vi "Encode_Base64 (SubVI).vi"(8 "error in (no error)":errorcluster, 11 "File Path":path=path "C:/Users/Voodoo/Desktop/loc_eps_3dcartrot.gif") -> (0 "error out":errorcluster, 3 "Base 64":string)   [LabVIEW 2016]
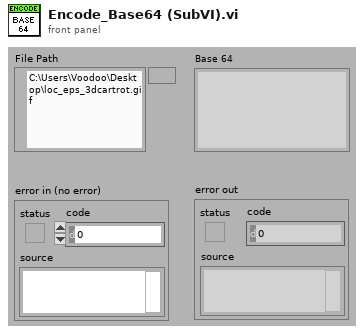
[diagram p1: front panel]
types:
  T1 = cluster{"unsigned byte array[0]":u8, "unsigned byte array[1]":u8, "unsigned byte array[2]":u8}
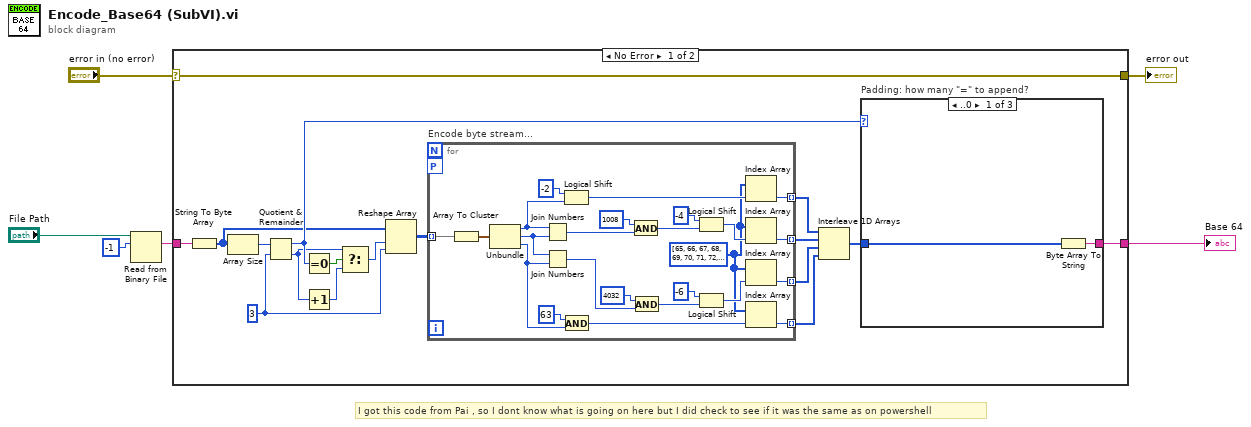
[diagram p0: block diagram]
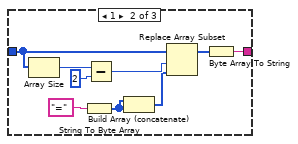
[diagram p2: hidden frame]
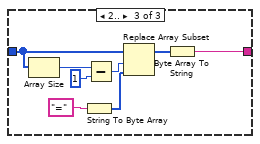
[diagram p3: hidden frame]
diagram:
  # "I got this code from Pai , so I dont know what is going on here but I did check to see if it was the same as on powershell"
  n1 = Read from Binary File(10:-1 ("count (1)"), 11:"File Path") -> (2:w1:string)  [unwired: 4 in, 3 out]
  n2 = case shown="No Error" "error in (no error)" {
    selector: "error in (no error)" -> [w23 w68]
    tunnel: w1 -> [w8 w67]
    tunnel: [w23 w68] -> w5
    tunnel: [w7 w67] -> w4
    frame No Error {
      w11 = 3 ("y")
      n3 = String To Byte Array(string=w8) -> (unsigned byte array=w12:u8[])
      n4 = Array Size(array=w12) -> (size(s)=w20:i32)
      n5 = Quotient & Remainder(x=w20, y=w11) -> (x-y*floor(x/y)=w21:i32, floor(x/y)=w14:i32)
      n6 = Equal To 0?(x=w21) -> (x = 0?=w22:bool)
      n7 = Increment(x=w14) -> (x+1=w15:i32)
      n8 = Select(t=w14, s=w22, f=w15) -> (s? t:f=w10:i32)
      n9 = Reshape Array(w12, w10, w11) -> (w9:u8[][])
      n10 = for "Encode byte stream..." {
        tunnel: [w26] -> w16 mode=indexing
        tunnel: [w27] -> w17 mode=indexing
        tunnel: [w28] -> w18 mode=indexing
        tunnel: [w29] -> w19 mode=indexing
        workers-P: _ -> [_]
        tunnel: w9 -> [w24] mode=indexing
        w25 = u8[] [65, 66, 67, 68, 69, 70, 71, 72, 73, 74, 75, 76, 77, 78, 79, 80, 81, 82, 83, 84, 85, 86, 87, 88, 89, 90, 97, 98, 99, 100, 101, 102, 103, 104, 105, 106, 107, 108, 109, 110, 111, 112, 113, 114, 115, 116, 117, 118, 119, 120, 121, 122, 48, 49, 50, 51, 52, 53, 54, 55, 56, 57, 43, 47] ("unsigned byte array")
        n11 = Array To Cluster(array=w24) -> (cluster=w47:T1)
        n12 = Unbundle(w47) -> ("unsigned byte array[0]"=w36:u8, "unsigned byte array[1]"=w41:u8, "unsigned byte array[2]"=w35:u8)
        n13 = Join Numbers(hi=w36, lo=w41) -> ((hi.lo)=w45:u16)
        n14 = Join Numbers(hi=w41, lo=w35) -> ((hi.lo)=w40:u16)
        n15 = Logical Shift(y=i8 -2, x=w36) -> (x << y=w33:u8)
        n16 = And(x=u8 63, y=w35) -> (x .and. y?=w30:u8)
        n17 = And(x=u16 1008, y=w45) -> (x .and. y?=w43:u16)
        n18 = And(x=u16 4032, y=w40) -> (x .and. y?=w38:u16)
        n19 = Logical Shift(y=i8 -4, x=w43) -> (x << y=w32:u16)
        n20 = Logical Shift(y=i8 -6, x=w38) -> (x << y=w31:u16)
        n21 = Index Array(array=w25, index=w33) -> (element=w29:u8)
        n22 = Index Array(array=w25, index=w32) -> (element=w28:u8)
        n23 = Index Array(array=w25, index=w31) -> (element=w27:u8)
        n24 = Index Array(array=w25, index=w30) -> (element=w26:u8)
      }
      n25 = Interleave 1D Arrays(w19, w18, w17, w16) -> (w13:u8[])
      n26 = case "Padding: how many \"=\" to append?" shown="..0" w21 {
        tunnel: [w48 w55 w63] -> w7
        tunnel: w13 -> [w49 w53 w61]
        frame ..0 {
          n27 = Byte Array To String(unsigned byte array=w49) -> (string=w48:string)
        }
        frame 1 {
          n28 = Array Size(array=w53) -> (size(s)=w54:i32)
          n29 = String To Byte Array(string="=") -> (unsigned byte array=w51:u8[])
          n30 = Subtract(x=w54, y=2) -> (x-y=w57:i32)
          n31 = Build Array (concatenate)(w51, w51) -> (w50:u8[])
          n32 = Replace Array Subset(array=w53, new element=w50, index=w57) -> (w56:u8[])
          n33 = Byte Array To String(unsigned byte array=w56) -> (string=w55:string)
        }
        frame 2.. {
          n34 = Array Size(array=w61) -> (size(s)=w62:i32)
          n35 = String To Byte Array(string="=") -> (unsigned byte array=w59:u8[])
          n36 = Subtract(x=w62, y=1) -> (x-y=w65:i32)
          n37 = Replace Array Subset(array=w61, new element=w59, index=w65) -> (w64:u8[])
          n38 = Byte Array To String(unsigned byte array=w64) -> (string=w63:string)
        }
      }
    }
    frame Error {
    }
  }
  "Base 64" <- w4
  "error out" <- w5
